vi "Write Beads to TDMS.vi"(9 "Bead Profiles":cluster{dbl[], dbl[]}[](array[cluster]), 10 "Layer #":i32, 11 "Refnum in":refnum<k34>) -> (3 "Refnum out":refnum<k34>)   [LabVIEW 2016]
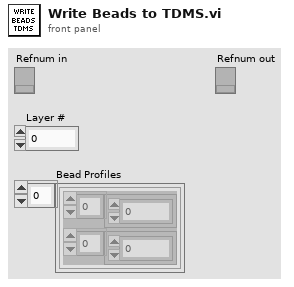
[diagram p1: front panel]
types:
  T1 = cluster{"Bead Profiles[0]":cluster{dbl[], dbl[]}, "Bead Profiles[1]":cluster{dbl[], dbl[]}, "Bead Profiles[2]":cluster{dbl[], dbl[]}, "Bead Profiles[3]":cluster{dbl[], dbl[]}, "Bead Profiles[4]":cluster{dbl[], dbl[]}}
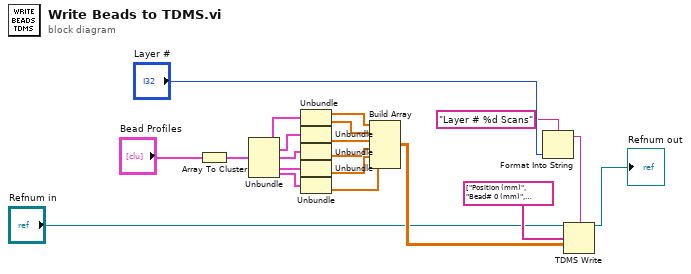
[diagram p0: block diagram]
diagram:
  n1 = Array To Cluster(array="Bead Profiles") -> (cluster=w6:T1)
  n2 = Unbundle(w6) -> ("Bead Profiles[0]"=w7:cluster{dbl[], dbl[]}, "Bead Profiles[1]"=w8:cluster{dbl[], dbl[]}, "Bead Profiles[2]"=w9:cluster{dbl[], dbl[]}, "Bead Profiles[3]"=w10:cluster{dbl[], dbl[]}, "Bead Profiles[4]"=w11:cluster{dbl[], dbl[]})
  n3 = Unbundle(w7) -> (w12:dbl[], w13:dbl[])
  n4 = Unbundle(w8) -> (w14:dbl[])  [unwired: 1 out]
  n5 = Unbundle(w9) -> (w15:dbl[])  [unwired: 1 out]
  n6 = Unbundle(w10) -> (w16:dbl[])  [unwired: 1 out]
  n7 = Unbundle(w11) -> (w17:dbl[])  [unwired: 1 out]
  n8 = Build Array(w12, w13, w14, w15, w16, w17) -> (w18:dbl[][])
  n9 = Format Into String(format string="Layer # %d Scans", "Layer #") -> (resulting string=w1:string)  [unwired: 2 in, 1 out]
  n10 = TDMS Write(0:"Refnum in", 5:w1, 7:string[] ["Position (mm)", "Bead# 0 (mm)", "Bead# 1 (mm)", "Bead# 2 (mm)", "Bead# 3 (mm)", "Bead# 4 (mm)"] ("channel name(s) in (Untitled)"), 9:w18) -> (4:→"Refnum out":refnum<k34>)  [unwired: 2 in, 3 out]
